vi "Shutdown.vi"(8 "error in (no error)":errorcluster, 9 "Pound":refnum<class "Pound.lvclass">, 10 "restart system":bool, 11 "Qbus in":refnum<class "Qbus.lvclass">) -> (0 "error out":errorcluster)   [LabVIEW 2017]
uses:
  <vilib>/addons/Qbus/Qbus.lvclass
  <vilib>/NI/Software Watchdog/Pound/Pound.lvclass
  <vilib>/addons/SystemInfoProcess/SystemInfoProcess.lvlib
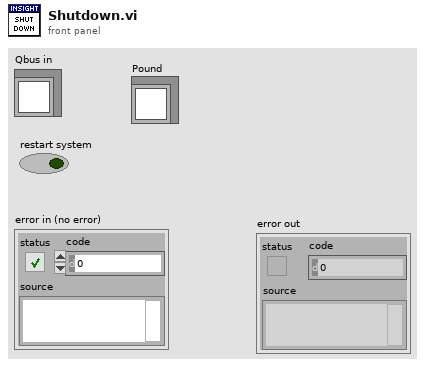
[diagram p1: front panel]
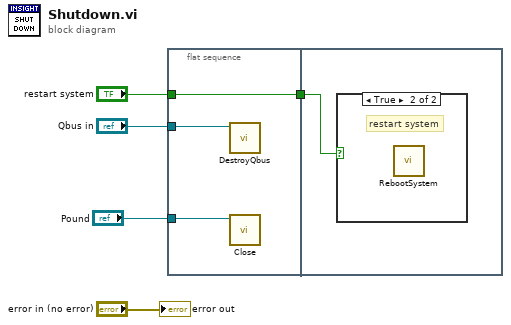
[diagram p0: block diagram]
diagram:
  n1 = flat-sequence {
    tunnel: [w7] -> w4
    tunnel: "Qbus in" -> [w8]
    tunnel: "restart system" -> [w7]
    tunnel: "Pound" -> [w6]
    tunnel: w4 -> [w9]
    frame #0 {
      n2 = call <vilib>:"DestroyQbus.vi"("Qbus"=w8) -> ()  [unwired: 10 in, 1 out]
      n3 = call <vilib>:"Close.vi"("Pound"=w6) -> ()  [unwired: 10 in, 1 out]
    }
    frame #1 {
      n4 = case shown="True" w9 {
        frame False {
        }
        frame True {
          # "restart system"
          n5 = call <vilib>:"RebootSystem.vi"() -> ()  [unwired: 11 in, 1 out]
        }
      }
    }
  }
  "error out" <- "error in (no error)"
